vi "apply control changes.vi"(6 "Prompt?":bool, 9 "new":string[][](array[string]), 10 "old":string[][](array[string]), 11 "dataset in":string[][][](array[string])) -> (2 "adjust all?":bool, 3 "dataset out":string[][][](array[string]))   [LabVIEW 2013, in "update vi properties.lvlib"]
uses:
  update vi properties.lvlib
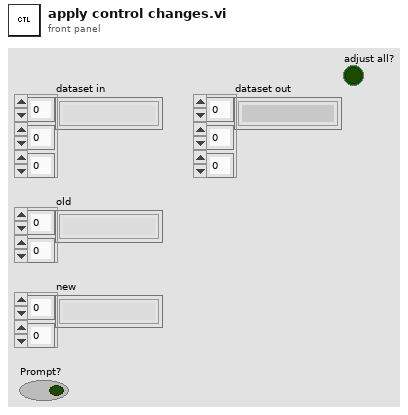
[diagram p1: front panel]
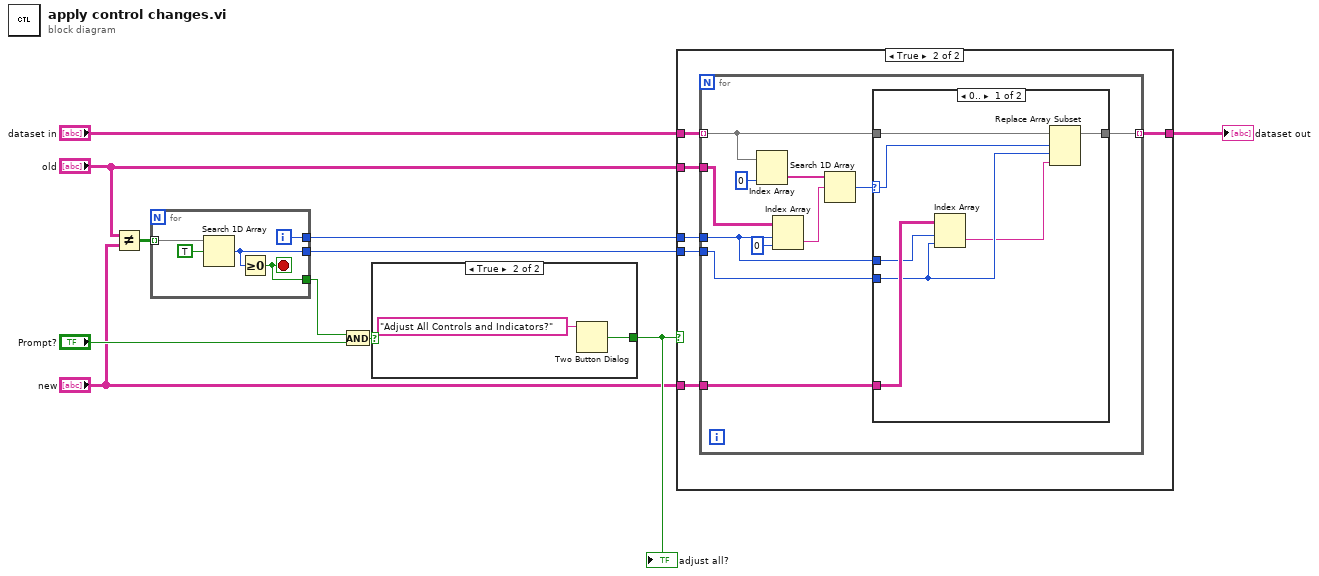
[diagram p0: block diagram]
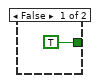
[diagram p4: hidden frame]
diagram:
  n1 = Not Equal?(x="old", y="new") -> (x != y?=w11:bool[][])
  n2 = for {
    tunnel: w11 -> [w16] mode=indexing
    tunnel: [w14] -> w2
    tunnel: [w13] -> w3
    tunnel: [w12] -> w10
    i -> [w13]
    stop <- w12 stop-if-true
    n3 = Search 1D Array(1D array=w16, element=TRUE) -> (index of element=w14:i32)  [unwired: 1 in]
    n4 = Greater Or Equal To 0?(x=w14) -> (x >= 0?=w12:bool)
  }
  n5 = And(x=w10, y="Prompt?") -> (x .and. y?=w8:bool)
  n6 = case shown="True" w8 {
    tunnel: [TRUE w18] -> w7
    frame False {
    }
    frame True {
      n7 = Two Button Dialog(message="Adjust All Controls and Indicators?") -> (T button?=w18:bool)  [unwired: 2 in]
    }
  }
  "adjust all?" <- w7
  n8 = case shown="True" w7 {
    tunnel: "dataset in" -> [w20 w26]
    tunnel: [w20 w22] -> w5
    tunnel: "old" -> [_ w25]
    tunnel: w3 -> [_ w24]
    tunnel: w2 -> [_ w23]
    tunnel: "new" -> [_ w21]
    frame False {
    }
    frame True {
      n9 = for {
        tunnel: w26 -> [w32] mode=indexing
        tunnel: w25 -> [w35]
        tunnel: w24 -> [w27]
        tunnel: w23 -> [w29]
        tunnel: [w30] -> w22 mode=indexing
        tunnel: w21 -> [w28]
        n10 = Index Array(array=w32, index (col)=0 ("disabled index (col)")) -> (element=w34:string[])  [unwired: 1 in]
        n11 = Index Array(array=w35, index (row)=w27, index (col)=0 ("disabled index (col)")) -> (element=w33:string)
        n12 = Search 1D Array(1D array=w34, element=w33) -> (index of element=w31:i32)  [unwired: 1 in]
        n13 = case shown="0.." w31 {
          selector: w31 -> [w42 _]
          tunnel: w32 -> [w44 w45]
          tunnel: [w43 w45] -> w30
          tunnel: w29 -> [w39 _]
          tunnel: w28 -> [w41 _]
          tunnel: w27 -> [w40 _]
          frame 0.. {
            n14 = Index Array(array=w41, index (row)=w40, index (col)=w39) -> (element=w38:string)
            n15 = Replace Array Subset(array=w44, new element=w38, index (row)=w42, index (col)=w39) -> (w43:string[][])
          }
          frame ..-1 {
          }
        }
      }
    }
  }
  "dataset out" <- w5
